vi "VLC Video Stream handler.vi"(7 "CameraArray":refnum<vi>, 8 "Exit":refnum<vi>, 10 "Video Feed 2":refnum<vi>, 11 "Camera 1":refnum<k24>(container)) -> (0 "error out":errorcluster)   [LabVIEW 2017]
uses:
  System.Windows.Forms
panel:
  in  "path in":path=path "C:/Program Files (x86)/VideoLAN/VLC/libvlc.dll"
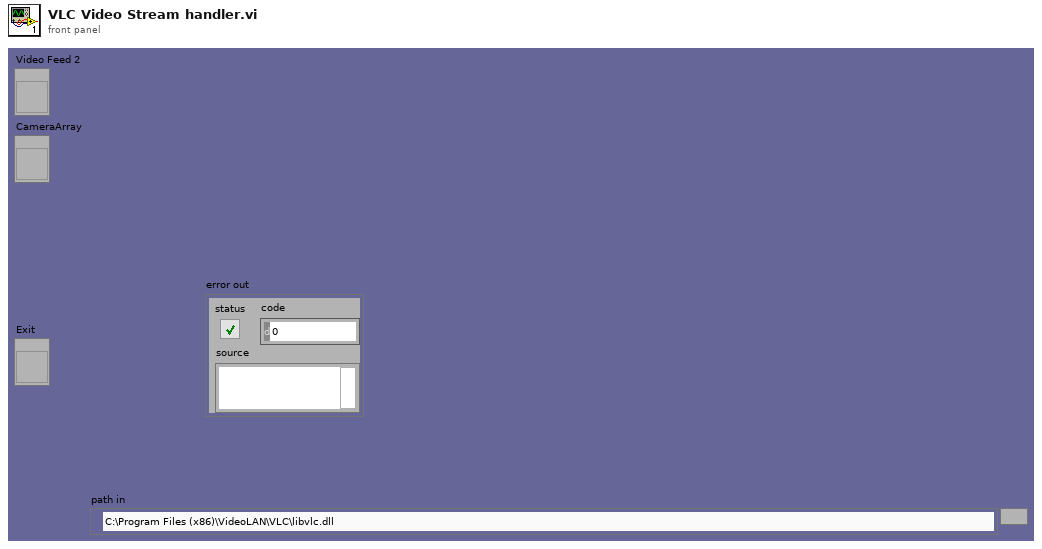
[diagram p1: front panel]
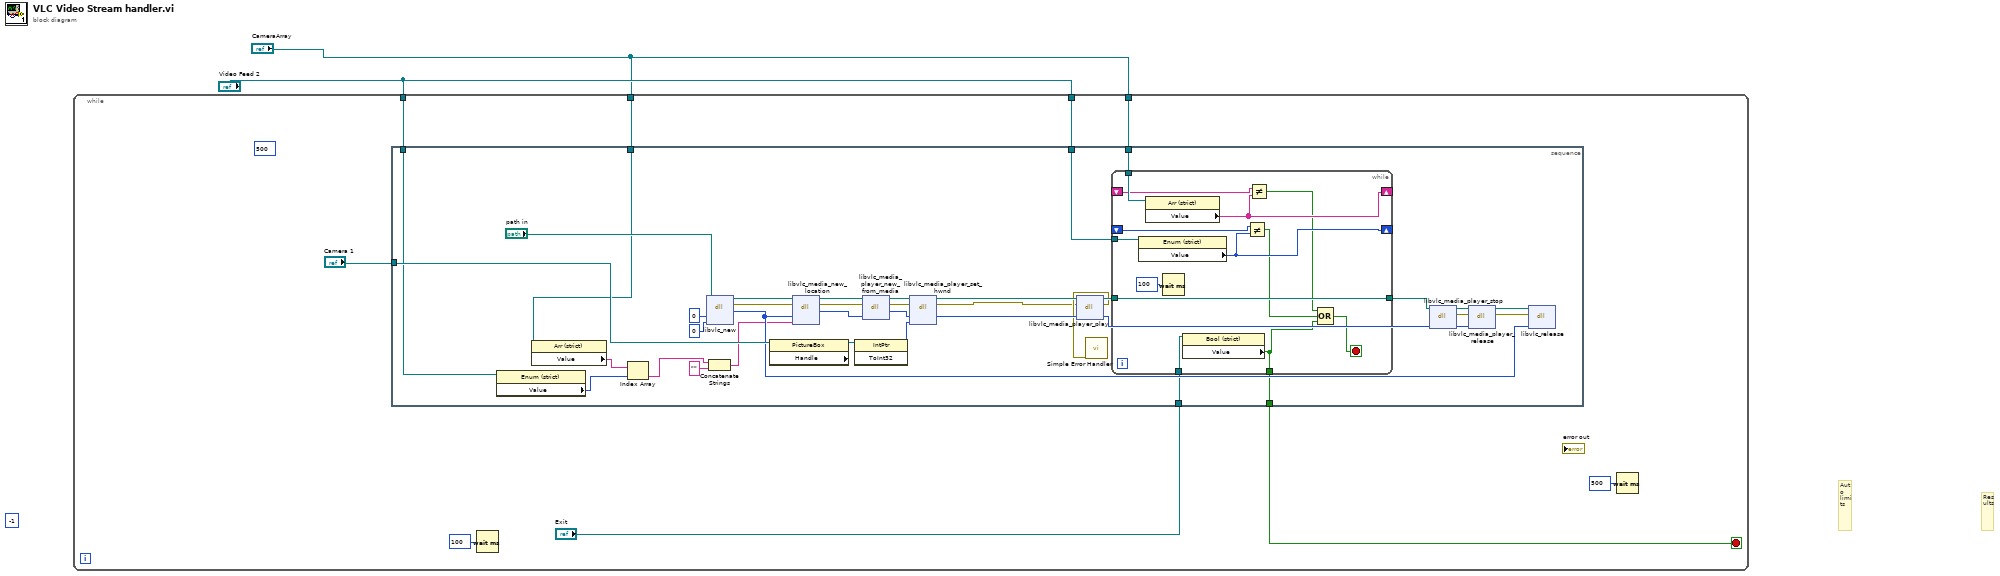
[diagram p0: block diagram]
diagram:
  (unwired) -1
  # "Results"
  # "Auto limits"
  n1 = while {
    tunnel: "Video Feed 2" -> [w8]
    tunnel: "CameraArray" -> [w7]
    tunnel: "Video Feed 2" -> [w4]
    tunnel: "CameraArray" -> [w3]
    stop <- w5 stop-if-true
    (unwired) 500
    n2 = stacked-sequence {
      tunnel: "Camera 1" -> [w49]
      tunnel: w8 -> [w22]
      tunnel: w7 -> [w21]
      tunnel: "Exit" -> [w20]
      tunnel: [w19] -> w5
      tunnel: w4 -> [w17]
      tunnel: w3 -> [w14]
      frame #0 {
        n3 = property class="Enum (strict)"(reference=w17) -> ("Value"=w16:enum16{"Camera 1", "Camera2", "Mobile"})  [unwired: 1 in, 2 out]
        n4 = property class="Arr (strict)"(reference=w14) -> ("Value"=w18:string[])  [unwired: 1 in, 2 out]
        n5 = Index Array(array=w18, index=w16) -> (element=w15:string)
        n6 = dll-call lib="C:/Program Files (x86)/VideoLAN/VLC/libvlc.dll" fn="libvlc_new"(path in="path in", "argc"=i16 0, "argv"=u8 0) -> (path out=w28:path, error out=w31:errorcluster, "return type"=w40:i32)  [unwired: 4 in]
        n7 = Concatenate Strings(w15, "" ("string")) -> (w37:string)
        n8 = property class="PictureBox"(reference=w49) -> ("Handle"=w24:refnum<k24>)  [unwired: 1 in, 2 out]
        n9 = dll-call lib="C:/Program Files (x86)/VideoLAN/VLC/libvlc.dll" fn="libvlc_media_new_location"(path in=w28, error in=w31, "p_instance"=w40, "path"=w37) -> (path out=w25:path, error out=w36:errorcluster, "return type"=w35:i32)  [unwired: 3 in]
        n10 = invoke class="IntPtr" method="ToInt32"(reference=w24) -> ("ToInt32"=w23:i32)  [unwired: 2 in, 2 out]
        n11 = dll-call lib="C:/Program Files (x86)/VideoLAN/VLC/libvlc.dll" fn="libvlc_media_player_new_from_media"(path in=w25, error in=w36, "p_md"=w35) -> (path out=w27:path, error out=w34:errorcluster, "return type"=w32:i32)  [unwired: 2 in]
        n12 = dll-call lib="C:/Program Files (x86)/VideoLAN/VLC/libvlc.dll" fn="libvlc_media_player_set_hwnd"(path in=w27, error in=w34, "p_mi"=w32, "drawable"=w23) -> (path out=w26:path, error out=w12:errorcluster, "p_mi"=w33:i32)  [unwired: 3 in]
        n13 = dll-call lib="C:/Program Files (x86)/VideoLAN/VLC/libvlc.dll" fn="libvlc_media_player_play"(path in=w26, error in=w12, "p_mi"=w33) -> (path out=w46:path, error out=w13:errorcluster, "p_mi"=w39:i32)  [unwired: 2 in]
        n14 = call <vilib>:"Simple Error Handler.vi"("error in (no error)"=w13) -> ()  [unwired: 4 in, 5 out]
        n15 = while {
          tunnel: w46 -> [w61]
          tunnel: [w61] -> w47
          shift-right: [w57] -> _
          shift-left: _ -> [w58]
          shift-right: [w55] -> _
          shift-left: _ -> [w56]
          tunnel: w22 -> [w60]
          tunnel: w21 -> [w59]
          tunnel: w20 -> [w54]
          tunnel: [w51] -> w19
          stop <- w50 stop-if-true
          n16 = property class="Enum (strict)"(reference=w60) -> ("Value"=w55:enum16{"Camera 1", "Camera2", "Mobile"})  [unwired: 1 in, 2 out]
          n17 = property class="Arr (strict)"(reference=w59) -> ("Value"=w57:string[])  [unwired: 1 in, 2 out]
          n18 = Wait (ms)(milliseconds to wait=u32 100) -> ()  [unwired: 1 out]
          n19 = property class="Bool (strict)"(reference=w54) -> ("Value"=w51:bool)  [unwired: 1 in, 2 out]
          n20 = Not Equal?(x=w56, y=w55) -> (x != y?=w52:bool)
          n21 = Not Equal?(x=w58, y=w57) -> (x != y?=w53:bool)
          n22 = Compound Arithmetic op=OR(w53, w52, w51) -> (w50:bool)
        }
        n23 = dll-call lib="C:/Program Files (x86)/VideoLAN/VLC/libvlc.dll" fn="libvlc_media_player_stop"(path in=w47, "p_mi"=w39) -> (path out=w42:path, error out=w45:errorcluster, "p_mi"=w44:i32)  [unwired: 3 in]
        n24 = dll-call lib="C:/Program Files (x86)/VideoLAN/VLC/libvlc.dll" fn="libvlc_media_player_release"(path in=w42, error in=w45, "p_mi"=w44) -> (path out=w41:path, error out=w43:errorcluster)  [unwired: 3 in]
        n25 = dll-call lib="C:/Program Files (x86)/VideoLAN/VLC/libvlc.dll" fn="libvlc_release"(path in=w41, error in=w43, "p_instnace"=w40) -> ()  [unwired: 3 in, 2 out]
      }
    }
    n26 = Wait (ms)(milliseconds to wait=u32 100) -> ()  [unwired: 1 out]
    n27 = Wait (ms)(milliseconds to wait=u32 500) -> ()  [unwired: 1 out]
  }
